vi "servo_motor.vi"(8 "Duty Cycle":dbl(knob)=50.0 scale=3.0..10.0, 10 "Error In":errorcluster caption="Error In (no error)", 11 "Enable Outputs":bool=TRUE) -> (3 "error out":errorcluster)   [LabVIEW 2016]
uses:
  <vilib>/DigilentWF/DigilentWF.lvlib
panel:
  # "The Duty cycle in term of percentage between 1 t o 2ms.\nThe Enable outputs switch to enable the servo motor."
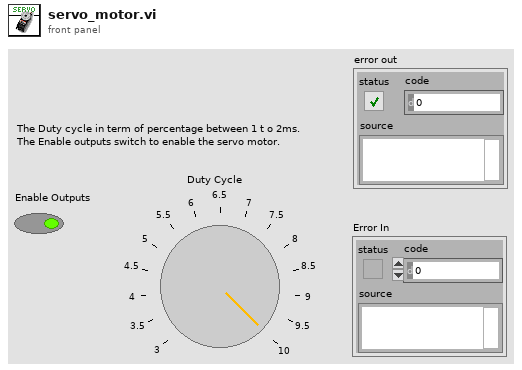
[diagram p1: front panel]
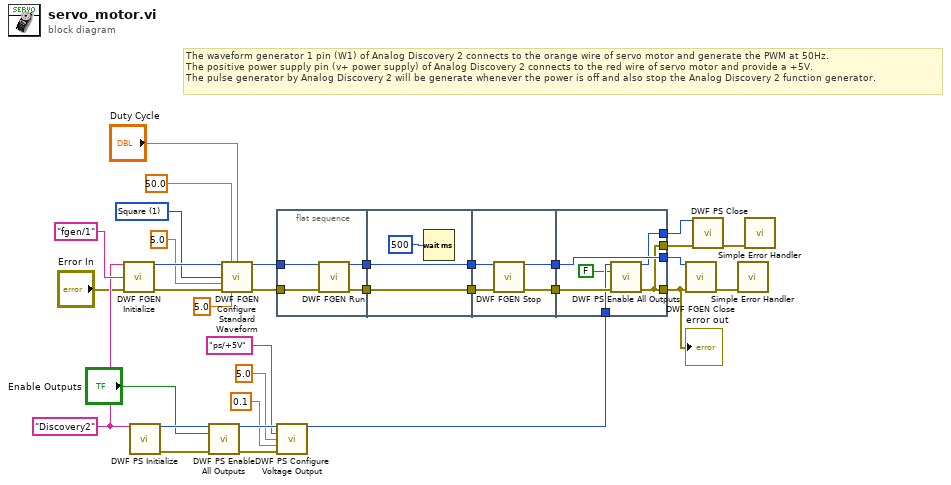
[diagram p0: block diagram]
diagram:
  w19 = 1 items=["Sine", "Square", "Triangle/Ramp", "DC"] ("Waveform Function")
  w32 = "Discovery2" ("Device Name")
  # "The waveform generator 1 pin (W1) of Analog Discovery 2 connects to the orange wire of servo motor and generate the PWM at 50Hz.\nThe positive power supply pin (v+ power supply) of Analog Discovery 2 connects to the red wire of servo motor and provide a +5V.\nThe pulse generator by Analog Discovery 2 will be generate whenever the power is off and also stop the Analog Discovery 2 function generator."
  n1 = call <vilib>:"DWF FGEN Initialize.vi"("Device Name"=w32, "Channel"="fgen/1", "Error In"="Error In") -> ("Instrument Handle Out"=w31:u32, "Error Out"=w30:errorcluster)  [unwired: 11 in]
  n2 = call <vilib>:"DWF PS Initialize.vi"("Device Name"=w32) -> ("Instrument Handle Out"=w21:u32, "Error Out"=w20:errorcluster)  [unwired: 13 in]
  n3 = call <vilib>:"DWF PS Enable All Outputs.vi"("Instrument Handle In"=w21, "Enable Outputs"="Enable Outputs", "Error In"=w20) -> ("Instrument Handle Out"=w13:u32, "Error Out"=w12:errorcluster)  [unwired: 11 in]
  n4 = call <vilib>:"DWF FGEN Configure Standard Waveform.vi"("Instrument Handle In"=w31, "Frequency"=50.0, "Duty Cycle"="Duty Cycle", "Waveform Function"=w19, "Amplitude"=5.0, "Error In"=w30, "DC Offset"=5.0) -> ("Instrument Handle Out"=w8:u32, "Error Out"=w7:errorcluster)  [unwired: 7 in]
  n5 = flat-sequence {
    tunnel: [w35] -> w27
    tunnel: [w36] -> w26
    tunnel: w8 -> [w37]
    tunnel: w7 -> [w34]
    tunnel: [w40] -> w25
    tunnel: [w39] -> w24
    tunnel: w27 -> [w39]
    tunnel: w26 -> [w40]
    tunnel: w25 -> [w44]
    tunnel: w24 -> [w43]
    tunnel: [w42] -> w23
    tunnel: [w41] -> w22
    tunnel: [w46] -> w28
    tunnel: [w50] -> w29
    tunnel: w23 -> [w50]
    tunnel: w22 -> [w49]
    tunnel: w5 -> [w48]
    tunnel: [w47] -> w3
    tunnel: [w46] -> w2
    frame #0 {
      n6 = call <vilib>:"DWF FGEN Run.vi"("Instrument Handle In"=w37, "Error In"=w34) -> ("Instrument Handle Out"=w36:u32, "Error Out"=w35:errorcluster)  [unwired: 12 in]
    }
    frame #1 {
      n7 = Wait (ms)(milliseconds to wait=u32 500) -> ()  [unwired: 1 out]
    }
    frame #2 {
      n8 = call <vilib>:"DWF FGEN Stop.vi"("Instrument Handle In"=w44, "Error In"=w43) -> ("Instrument Handle Out"=w42:u32, "Error Out"=w41:errorcluster)  [unwired: 12 in]
    }
    frame #3 {
      n9 = call <vilib>:"DWF PS Enable All Outputs.vi"("Instrument Handle In"=w48, "Enable Outputs"=FALSE, "Error In"=w49) -> ("Instrument Handle Out"=w47:u32, "Error Out"=w46:errorcluster)  [unwired: 11 in]
    }
  }
  n10 = call <vilib>:"DWF PS Configure Voltage Output.vi"("Instrument Handle In"=w13, "Channel"="ps/+5V", "Voltage Level"=5.0, "Current Limit"=0.1, "Error In"=w12) -> ("Instrument Handle Out"=w5:u32)  [unwired: 9 in, 1 out]
  n11 = call <vilib>:"DWF FGEN Close.vi"("Instrument Handle In"=w29, "Error In"=w28) -> ("Error Out"=w1:errorcluster)  [unwired: 13 in]
  n12 = call <vilib>:"DWF PS Close.vi"("Instrument Handle In"=w3, "Error In"=w2) -> ("Error Out"=w4:errorcluster)  [unwired: 13 in]
  n13 = call <vilib>:"Simple Error Handler.vi"("error in (no error)"=w1) -> ()  [unwired: 4 in, 5 out]
  n14 = call <vilib>:"Simple Error Handler.vi"("error in (no error)"=w4) -> ()  [unwired: 4 in, 5 out]
  "error out" <- w28
